vi "MeasLeakRate12.vi"() -> ()   [LabVIEW 2011]
panel:
  out "Angle(deg)":string
  out "error out":errorcluster
  out "fit":cluster{"element":dbl, "Value":dbl}[](array[cluster])
  out "T-T0,P":cluster{"element":dbl, "element":dbl}[](array[cluster])
  out "t0":dbl format="%#_8f"
  out "XY Graph":T1(graph)
  out "S00":i32
  out "S20":dbl
  out "S11":dbl
  out "S10":dbl
  out "S01":dbl
  out "T,P":cluster{"element":dbl, "element":dbl}[](array[cluster])
  out "dPdt":dbl
  out "P0":dbl
  out "average P (Torr)":string
  in  "Control Valve local":bool
  in  "Exhaust Local":bool
  in  "Exhaust Close":bool
  in  "Exhaust Open":bool
  in  "Control Close":bool
  in  "Control Open":bool
  in  "reset":bool
  in  "# points to watch":i32=60
  out "leak rate (Torr/min)":string
  out "P":dbl
  out "first":bool=TRUE
  in  "interval (s)":dbl=0.5
  in  "stop":bool
  out "P(Torr)":string
  # "Pressure control valve:"
  # "Exahaust valve:"
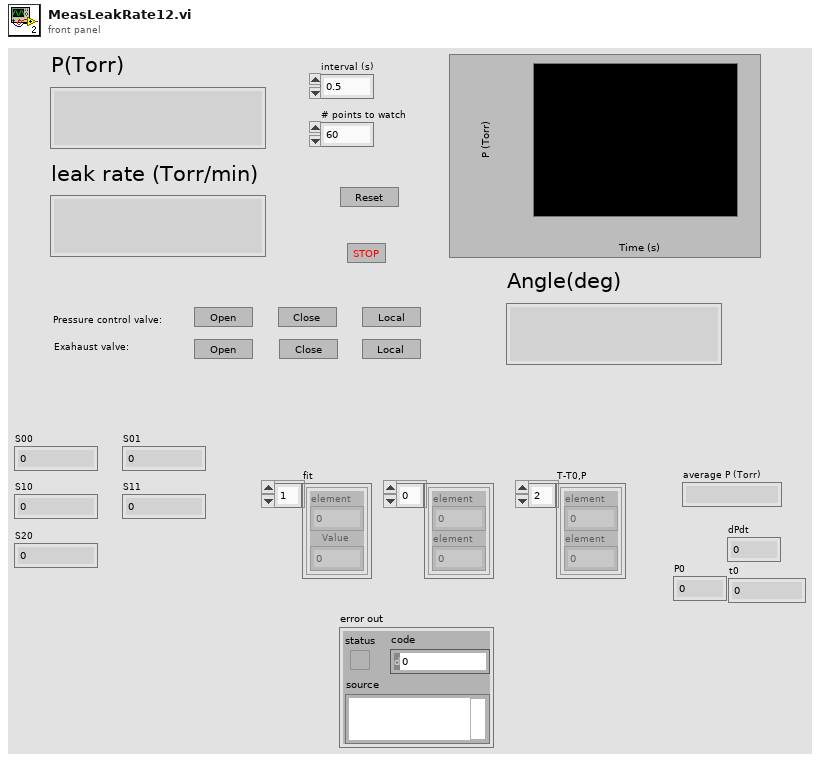
[diagram p1: front panel]
types:
  T1 = cluster{"Value":cluster{"element":dbl, "element":dbl}[]}[]
  T2 = cluster{"Value":cluster{"element":dbl, "Value":dbl}[]}[]
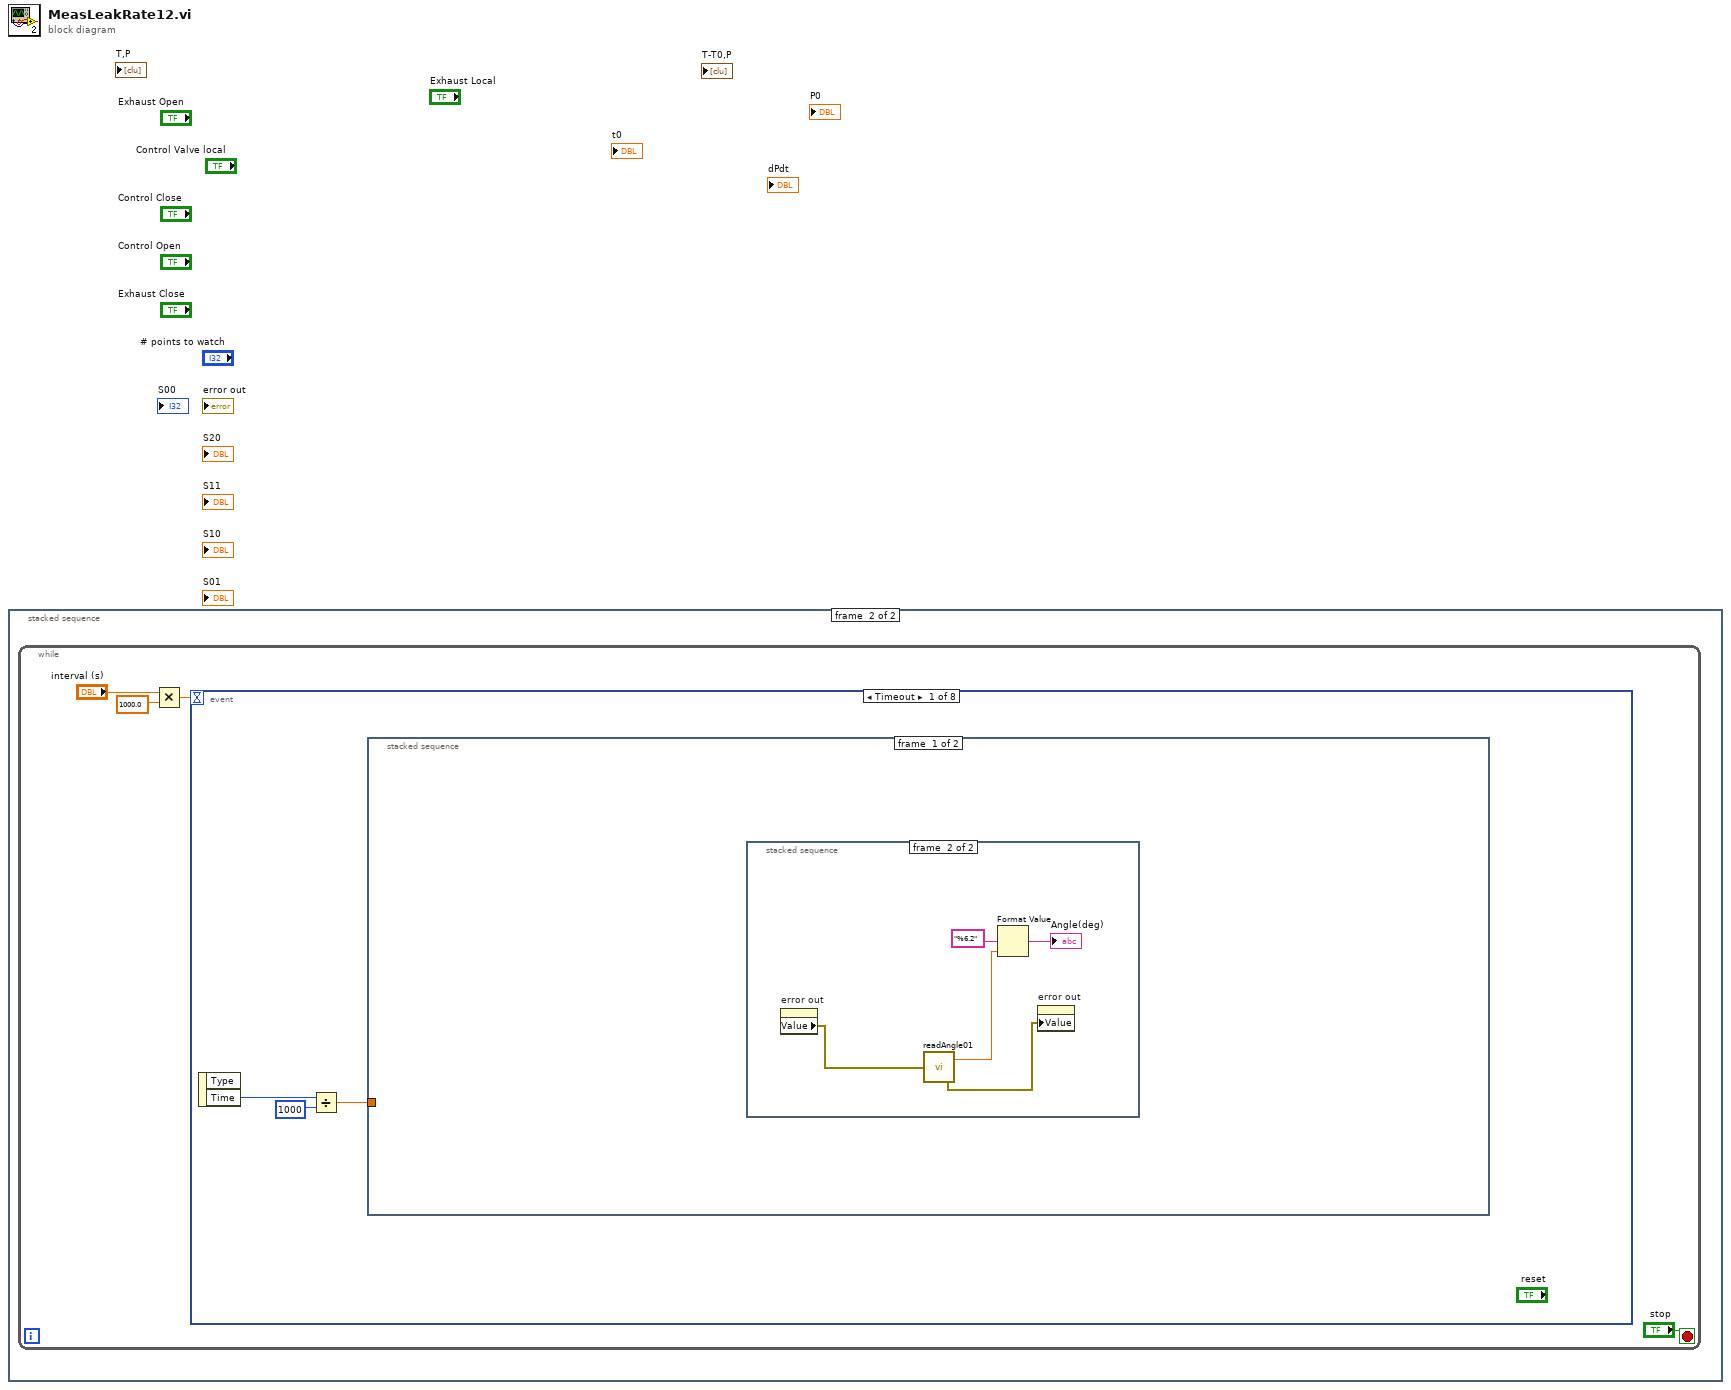
[diagram p0: block diagram]
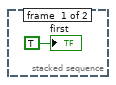
[diagram p2: hidden frame]
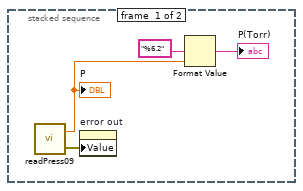
[diagram p3: hidden frame]
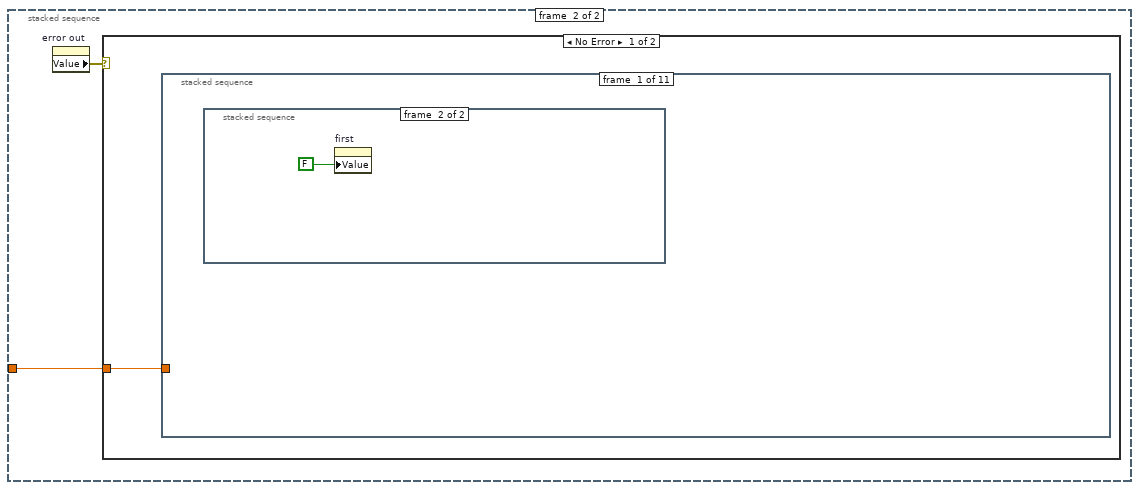
[diagram p4: hidden frame]
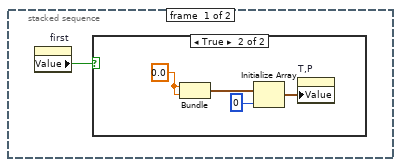
[diagram p5: hidden frame]
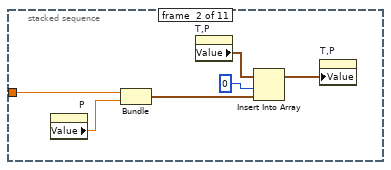
[diagram p7: hidden frame]
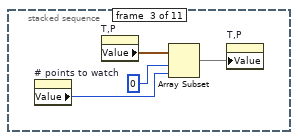
[diagram p8: hidden frame]
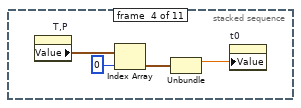
[diagram p9: hidden frame]
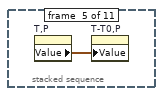
[diagram p10: hidden frame]
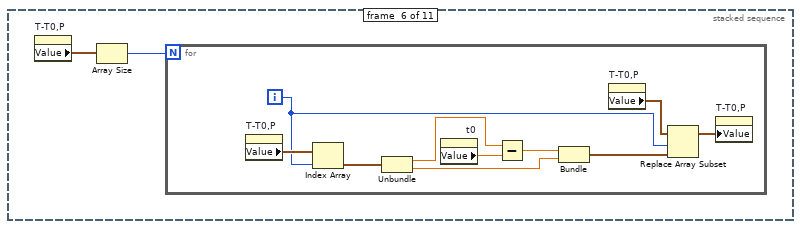
[diagram p11: hidden frame]
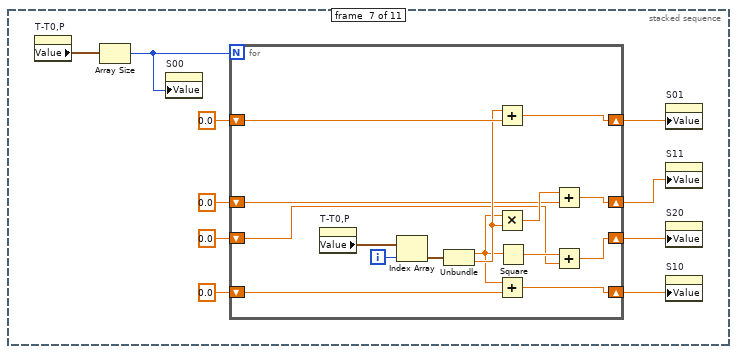
[diagram p12: hidden frame]
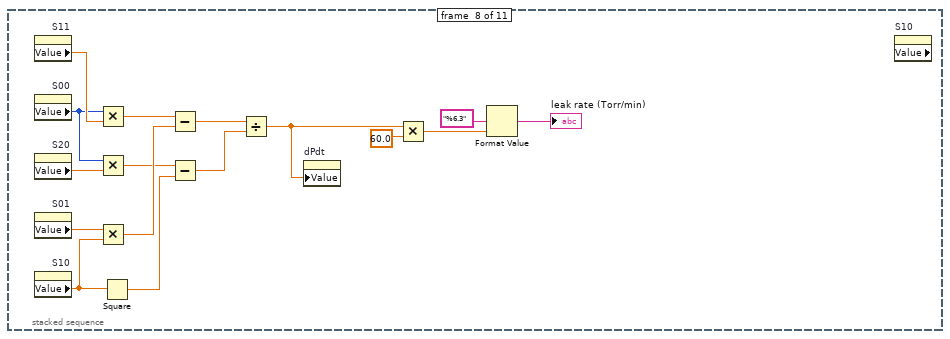
[diagram p13: hidden frame]
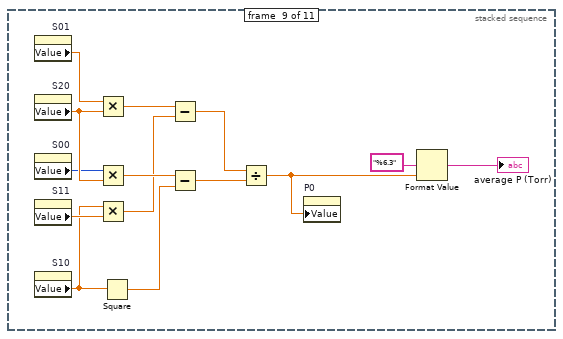
[diagram p14: hidden frame]
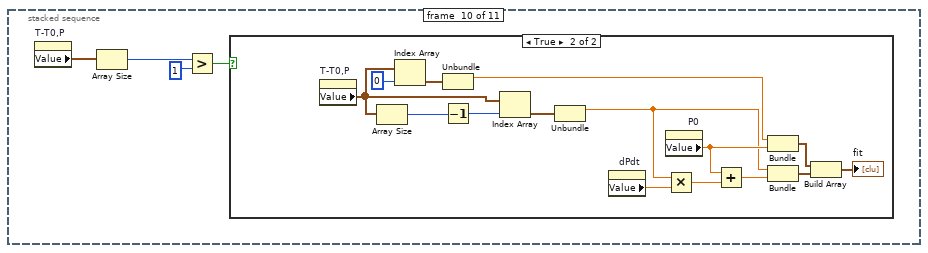
[diagram p15: hidden frame]
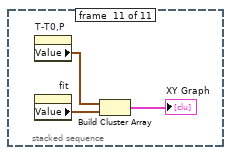
[diagram p17: hidden frame]
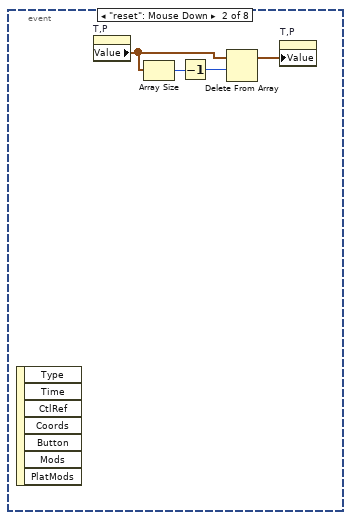
[diagram p19: hidden frame]
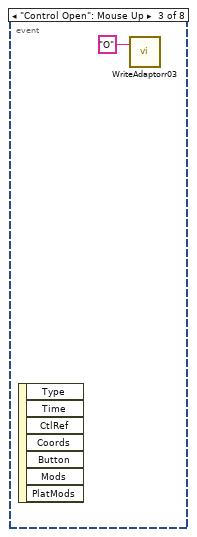
[diagram p20: hidden frame]
diagram:
  n1 = stacked-sequence {
    frame #0 {
      "first" <- TRUE ("first")
    }
    frame #1 {
      n2 = while {
        stop <- "stop" stop-if-true
        n3 = Multiply(x="interval (s)", y=1000.0) -> (x*y=w3:dbl)
        n4 = event shown="[0] Timeout" {
          selector: _ -> [_ _ _ _ _ _ _ _]
          dyn-events: _ -> [_ _ _ _ _ _ _ _]
          timeout: w3 -> [_ _ _ _ _ _ _ _]
          event Timeout {
            n5 = event-data() -> ("Time"=w8:u32)  [unwired: 1 in, 1 out]
            n6 = Divide(x=w8, y=u32 1000) -> (x/y=w6:dbl)
            n7 = stacked-sequence {
              tunnel: w6 -> [_ w18]
              frame #0 {
                n8 = stacked-sequence {
                  frame #0 {
                    n9 = call "readPress09.vi"() -> ("P"=w11:dbl, "error out"=w9:errorcluster)  [unwired: 1 in]
                    "P" <- w11
                    n10 = property on="error out" class="Clust (strict)"("Value"=w9) -> ()  [unwired: 2 in, 2 out]
                    n11 = Format Value(format string="%6.2", value (0)=w11) -> (output string=→"P(Torr)":string)  [unwired: 1 in]
                  }
                  frame #1 {
                    n12 = property on="error out" class="Clust (strict)"() -> ("Value"=w13:errorcluster)  [unwired: 2 in, 2 out]
                    n13 = call "readAngle01.vi"("error in"=w13) -> ("angle"=w14:dbl, "error out"=w15:errorcluster)
                    n14 = Format Value(format string="%6.2", value (0)=w14) -> (output string=→"Angle(deg)":string)  [unwired: 1 in]
                    n15 = property on="error out" class="Clust (strict)"("Value"=w15) -> ()  [unwired: 2 in, 2 out]
                  }
                }
              }
              frame #1 {
                n16 = property on="error out" class="Clust (strict)"() -> ("Value"=w19:errorcluster)  [unwired: 2 in, 2 out]
                n17 = case shown="No Error" w19 {
                  tunnel: w18 -> [w20 _]
                  frame No Error {
                    n18 = stacked-sequence {
                      tunnel: w20 -> [_ w27 _ _ _ _ _ _ _ _ _]
                      frame #0 {
                        n19 = stacked-sequence {
                          frame #0 {
                            n20 = property on="first" class="Bool (strict)"() -> ("Value"=w21:bool)  [unwired: 2 in, 2 out]
                            n21 = case shown="True" w21 {
                              frame False {
                              }
                              frame True {
                                w24 = 0.0 ("element")
                                n22 = Bundle("element"=w24, "element"=w24) -> (w23:cluster{"element":dbl, "element":dbl})  [unwired: 1 in]
                                n23 = Initialize Array(w23, 0 ("dimension size")) -> (w22:cluster{"element":dbl, "element":dbl}[])
                                n24 = property on="T,P" class="Arr (strict)"("Value"=w22) -> ()  [unwired: 2 in, 2 out]
                              }
                            }
                          }
                          frame #1 {
                            n25 = property on="first" class="Bool (strict)"("Value"=FALSE ("first")) -> ()  [unwired: 2 in, 2 out]
                          }
                        }
                      }
                      frame #1 {
                        n26 = property on="P" class="DigNum (strict)"() -> ("Value"=w32:dbl)  [unwired: 2 in, 2 out]
                        n27 = Bundle(w27, "Value"=w32) -> (w30:cluster{dbl, "Value":dbl})  [unwired: 1 in]
                        n28 = property on="T,P" class="Arr (strict)"() -> ("Value"=w31:cluster{"element":dbl, "element":dbl}[])  [unwired: 2 in, 2 out]
                        n29 = Insert Into Array(array=w31, index=0, new element=w30) -> (w28:cluster{"element":dbl, "element":dbl}[])
                        n30 = property on="T,P" class="Arr (strict)"("Value"=w28) -> ()  [unwired: 2 in, 2 out]
                      }
                      frame #2 {
                        n31 = property on="# points to watch" class="DigNum (strict)"() -> ("Value"=w34:i32)  [unwired: 2 in, 2 out]
                        n32 = property on="T,P" class="Arr (strict)"() -> ("Value"=w35:cluster{"element":dbl, "element":dbl}[])  [unwired: 2 in, 2 out]
                        n33 = Array Subset(array=w35, index=0, length=w34) -> (w33:cluster{"element":dbl, "element":dbl}[])
                        n34 = property on="T,P" class="Arr (strict)"("Value"=w33) -> ()  [unwired: 2 in, 2 out]
                      }
                      frame #3 {
                        n35 = property on="T,P" class="Arr (strict)"() -> ("Value"=w40:cluster{"element":dbl, "element":dbl}[])  [unwired: 2 in, 2 out]
                        n36 = Index Array(array=w40, index=0) -> (element=w38:cluster{"element":dbl, "element":dbl})
                        n37 = Unbundle(w38) -> ("element"=w37:dbl)  [unwired: 1 out]
                        n38 = property on="t0" class="DigNum (strict)"("Value"=w37) -> ()  [unwired: 2 in, 2 out]
                      }
                      frame #4 {
                        n39 = property on="T,P" class="Arr (strict)"() -> ("Value"=w41:cluster{"element":dbl, "element":dbl}[])  [unwired: 2 in, 2 out]
                        n40 = property on="T-T0,P" class="Arr (strict)"("Value"=w41) -> ()  [unwired: 2 in, 2 out]
                      }
                      frame #5 {
                        n41 = property on="T-T0,P" class="Arr (strict)"() -> ("Value"=w43:cluster{"element":dbl, "element":dbl}[])  [unwired: 2 in, 2 out]
                        n42 = Array Size(array=w43) -> (size(s)=w42:i32)
                        n43 = for {
                          N: w42 -> [_]
                          i -> [w44]
                          n44 = property on="T-T0,P" class="Arr (strict)"() -> ("Value"=w48:cluster{"element":dbl, "element":dbl}[])  [unwired: 2 in, 2 out]
                          n45 = Index Array(array=w48, index=w44) -> (element=w53:cluster{"element":dbl, "element":dbl})
                          n46 = Unbundle(w53) -> ("element"=w52:dbl, "element"=w49:dbl)
                          n47 = property on="t0" class="DigNum (strict)"() -> ("Value"=w51:dbl)  [unwired: 2 in, 2 out]
                          n48 = Subtract(x=w52, y=w51) -> (x-y=w50:dbl)
                          n49 = Bundle(w50, "element"=w49) -> (w47:cluster{dbl, "element":dbl})  [unwired: 1 in]
                          n50 = property on="T-T0,P" class="Arr (strict)"() -> ("Value"=w46:cluster{"element":dbl, "element":dbl}[])  [unwired: 2 in, 2 out]
                          n51 = Replace Array Subset(array=w46, new element=w47, index=w44) -> (w45:cluster{"element":dbl, "element":dbl}[])
                          n52 = property on="T-T0,P" class="Arr (strict)"("Value"=w45) -> ()  [unwired: 2 in, 2 out]
                        }
                      }
                      frame #6 {
                        n53 = property on="T-T0,P" class="Arr (strict)"() -> ("Value"=w54:cluster{"element":dbl, "element":dbl}[])  [unwired: 2 in, 2 out]
                        n54 = Array Size(array=w54) -> (size(s)=w58:i32)
                        n55 = property on="S00" class="DigNum (strict)"("Value"=w58) -> ()  [unwired: 2 in, 2 out]
                        n56 = for {
                          N: w58 -> [_]
                          shift-right: [w76] -> w57
                          shift-left: 0.0 -> [w78]
                          shift-right: [w75] -> w61
                          shift-left: 0.0 -> [w74]
                          shift-right: [w71] -> w56
                          shift-left: 0.0 -> [w70]
                          shift-right: [w67] -> w55
                          shift-left: 0.0 -> [w66]
                          i -> [w65]
                          n57 = property on="T-T0,P" class="Arr (strict)"() -> ("Value"=w64:cluster{"element":dbl, "element":dbl}[])  [unwired: 2 in, 2 out]
                          n58 = Index Array(array=w64, index=w65) -> (element=w77:cluster{"element":dbl, "element":dbl})
                          n59 = Unbundle(w77) -> ("element"=w69:dbl, "element"=w73:dbl)
                          n60 = Add(x=w73, y=w74) -> (x+y=w75:dbl)
                          n61 = Multiply(x=w69, y=w73) -> (x*y=w72:dbl)
                          n62 = Add(x=w69, y=w78) -> (x+y=w76:dbl)
                          n63 = Square(x=w69) -> (x^2=w68:dbl)
                          n64 = Add(x=w72, y=w70) -> (x+y=w71:dbl)
                          n65 = Add(x=w68, y=w66) -> (x+y=w67:dbl)
                        }
                        n66 = property on="S01" class="DigNum (strict)"("Value"=w61) -> ()  [unwired: 2 in, 2 out]
                        n67 = property on="S11" class="DigNum (strict)"("Value"=w56) -> ()  [unwired: 2 in, 2 out]
                        n68 = property on="S20" class="DigNum (strict)"("Value"=w55) -> ()  [unwired: 2 in, 2 out]
                        n69 = property on="S10" class="DigNum (strict)"("Value"=w57) -> ()  [unwired: 2 in, 2 out]
                      }
                      frame #7 {
                        n70 = property on="S11" class="DigNum (strict)"() -> ("Value"=w83:dbl)  [unwired: 2 in, 2 out]
                        n71 = property on="S00" class="DigNum (strict)"() -> ("Value"=w81:i32)  [unwired: 2 in, 2 out]
                        n72 = property on="S20" class="DigNum (strict)"() -> ("Value"=w82:dbl)  [unwired: 2 in, 2 out]
                        n73 = property on="S01" class="DigNum (strict)"() -> ("Value"=w80:dbl)  [unwired: 2 in, 2 out]
                        n74 = property on="S10" class="DigNum (strict)"() -> ("Value"=w84:dbl)  [unwired: 2 in, 2 out]
                        n75 = Multiply(x=w81, y=w83) -> (x*y=w94:dbl)
                        n76 = Multiply(x=w81, y=w82) -> (x*y=w92:dbl)
                        n77 = Multiply(x=w80, y=w84) -> (x*y=w93:dbl)
                        n78 = Square(x=w84) -> (x^2=w91:dbl)
                        n79 = Subtract(x=w94, y=w93) -> (x-y=w90:dbl)
                        n80 = Subtract(x=w92, y=w91) -> (x-y=w89:dbl)
                        n81 = Divide(x=w90, y=w89) -> (x/y=w79:dbl)
                        n82 = property on="dPdt" class="DigNum (strict)"("Value"=w79) -> ()  [unwired: 2 in, 2 out]
                        n83 = Multiply(x=w79, y=60.0) -> (x*y=w85:dbl)
                        n84 = Format Value(format string="%6.3", value (0)=w85) -> (output string=→"leak rate (Torr/min)":string)  [unwired: 1 in]
                        n85 = property on="S10" class="DigNum (strict)" props=["Value"]() -> ()  [unwired: 2 in, 3 out]
                      }
                      frame #8 {
                        n86 = property on="S01" class="DigNum (strict)"() -> ("Value"=w108:dbl)  [unwired: 2 in, 2 out]
                        n87 = property on="S20" class="DigNum (strict)"() -> ("Value"=w105:dbl)  [unwired: 2 in, 2 out]
                        n88 = property on="S00" class="DigNum (strict)"() -> ("Value"=w104:i32)  [unwired: 2 in, 2 out]
                        n89 = property on="S11" class="DigNum (strict)"() -> ("Value"=w107:dbl)  [unwired: 2 in, 2 out]
                        n90 = property on="S10" class="DigNum (strict)"() -> ("Value"=w106:dbl)  [unwired: 2 in, 2 out]
                        n91 = Multiply(x=w108, y=w105) -> (x*y=w96:dbl)
                        n92 = Multiply(x=w104, y=w105) -> (x*y=w99:dbl)
                        n93 = Multiply(x=w106, y=w107) -> (x*y=w95:dbl)
                        n94 = Square(x=w106) -> (x^2=w98:dbl)
                        n95 = Subtract(x=w96, y=w95) -> (x-y=w103:dbl)
                        n96 = Subtract(x=w99, y=w98) -> (x-y=w97:dbl)
                        n97 = Divide(x=w103, y=w97) -> (x/y=w100:dbl)
                        n98 = property on="P0" class="DigNum (strict)"("Value"=w100) -> ()  [unwired: 2 in, 2 out]
                        n99 = Format Value(format string="%6.3", value (0)=w100) -> (output string=→"average P (Torr)":string)  [unwired: 1 in]
                      }
                      frame #9 {
                        n100 = property on="T-T0,P" class="Arr (strict)"() -> ("Value"=w112:cluster{"element":dbl, "element":dbl}[])  [unwired: 2 in, 2 out]
                        n101 = Array Size(array=w112) -> (size(s)=w111:i32)
                        n102 = Greater?(x=w111, y=1) -> (0:w109:bool)
                        n103 = case shown="True" w109 {
                          frame False {
                          }
                          frame True {
                            n104 = property on="T-T0,P" class="Arr (strict)"() -> ("Value"=w116:cluster{"element":dbl, "element":dbl}[])  [unwired: 2 in, 2 out]
                            n105 = Array Size(array=w116) -> (size(s)=w126:i32)
                            n106 = Index Array(array=w116, index=0) -> (element=w124:cluster{"element":dbl, "element":dbl})
                            n107 = Unbundle(w124) -> ("element"=w119:dbl)  [unwired: 1 out]
                            n108 = Decrement(x=w126) -> (x-1=w125:i32)
                            n109 = Index Array(array=w116, index=w125) -> (element=w123:cluster{"element":dbl, "element":dbl})
                            n110 = Unbundle(w123) -> ("element"=w117:dbl)  [unwired: 1 out]
                            n111 = property on="dPdt" class="DigNum (strict)"() -> ("Value"=w122:dbl)  [unwired: 2 in, 2 out]
                            n112 = property on="P0" class="DigNum (strict)"() -> ("Value"=w120:dbl)  [unwired: 2 in, 2 out]
                            n113 = Multiply(x=w117, y=w122) -> (x*y=w121:dbl)
                            n114 = Add(x=w120, y=w121) -> (x+y=w118:dbl)
                            n115 = Bundle("element"=w119, "Value"=w120) -> (w115:cluster{"element":dbl, "Value":dbl})  [unwired: 1 in]
                            n116 = Bundle("element"=w117, w118) -> (w114:cluster{"element":dbl, dbl})  [unwired: 1 in]
                            n117 = Build Array(w115, w114) -> (→"fit":cluster{"element":dbl, "Value":dbl}[])
                          }
                        }
                      }
                      frame #10 {
                        n118 = property on="T-T0,P" class="Arr (strict)"() -> ("Value"=w130:cluster{"element":dbl, "element":dbl}[])  [unwired: 2 in, 2 out]
                        n119 = property on="fit" class="Arr (strict)"() -> ("Value"=w128:cluster{"element":dbl, "Value":dbl}[])  [unwired: 2 in, 2 out]
                        n120 = Build Cluster Array(w130, w128) -> (→"XY Graph":T2)
                      }
                    }
                  }
                  frame Error {
                  }
                }
              }
            }
          }
          event "reset": Mouse Down {
            n121 = event-data() -> ()  [unwired: 1 in, 7 out]
            n122 = property on="T,P" class="Arr (strict)"() -> ("Value"=w132:cluster{"element":dbl, "element":dbl}[])  [unwired: 2 in, 2 out]
            n123 = Array Size(array=w132) -> (size(s)=w134:i32)
            n124 = Decrement(x=w134) -> (x-1=w133:i32)
            n125 = Delete From Array(array=w132, length=w133) -> (array with subset deleted=w131:cluster{"element":dbl, "element":dbl}[])  [unwired: 1 in, 1 out]
            n126 = property on="T,P" class="Arr (strict)"("Value"=w131) -> ()  [unwired: 2 in, 2 out]
          }
          event "Control Open": Mouse Up {
            n127 = event-data() -> ()  [unwired: 1 in, 7 out]
            n128 = call "WriteAdaptorr03.vi"("string to write"="O") -> ()  [unwired: 1 in, 1 out]
          }
          event "Control Close": Mouse Up {
            n129 = event-data() -> ()  [unwired: 1 in, 7 out]
            n130 = call "WriteAdaptorr03.vi"("string to write"="C") -> ()  [unwired: 1 in, 1 out]
          }
          event "Exhaust Open": Mouse Up {
            n131 = event-data() -> ()  [unwired: 1 in, 7 out]
            n132 = call "set_vacuum.vi"("Vac Remote"=TRUE, "Atm Exhaust"=FALSE, "Vac Exhaust"=TRUE) -> ()
          }
          event "Exhaust Close": Mouse Up {
            n133 = event-data() -> ()  [unwired: 1 in, 7 out]
            n134 = call "set_vacuum.vi"("Vac Remote"=TRUE, "Atm Exhaust"=FALSE, "Vac Exhaust"=FALSE) -> ()
          }
          event "Exhaust Local": Mouse Up {
            n135 = event-data() -> ()  [unwired: 1 in, 7 out]
            n136 = call "set_vacuum.vi"() -> ()  [unwired: 3 in]
          }
          event "Control Valve local": Mouse Down? {
            n137 = event-data() -> ()  [unwired: 1 in, 7 out]
            n138 = call "WriteAdaptorr03.vi"("string to write"="D5") -> ()  [unwired: 1 in, 1 out]
            n139 = event-data() -> ()  [unwired: 5 in, 1 out]
          }
        }
      }
    }
  }
